vi "gentec-SOLO_PE.Read.vi"(8 "error in (no error)":errorcluster, 11 "VISA Refnum in":refnum<visa-resource-name>) -> (0 "error out":errorcluster, 1 "Return Parameters":u32[](array[numeric]), 2 "Error":string, 3 "VISA Refnum out":refnum<visa-resource-name>, 4 "Timeout":bool)   [LabVIEW 2014, in "gentec-SOLO-PE - Driver.lvlib"]
doc: "This VI tries to read out everything."
uses:
  gentec-SOLO-PE - Driver.lvlib
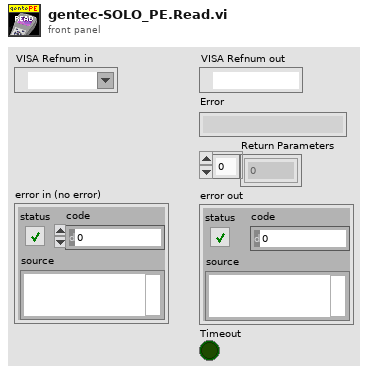
[diagram p1: front panel]
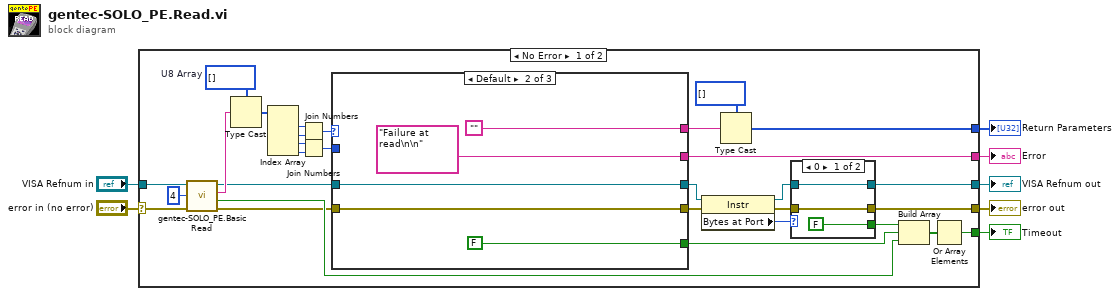
[diagram p0: block diagram]
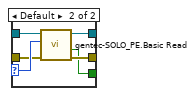
[diagram p2: hidden frame]
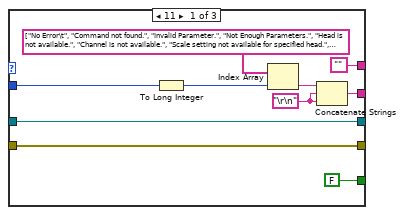
[diagram p3: hidden frame]
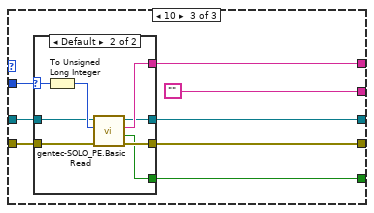
[diagram p4: hidden frame]
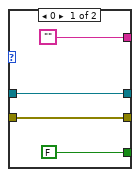
[diagram p5: hidden frame]
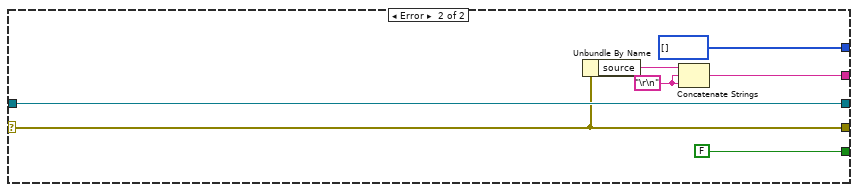
[diagram p6: hidden frame]
diagram:
  n1 = case shown="No Error" "error in (no error)" {
    selector: "error in (no error)" -> [w26 w85]
    tunnel: "VISA Refnum in" -> [w37 w86]
    tunnel: [w35 u32[] []] -> w6
    tunnel: [w19 w86] -> w5
    tunnel: [w12 w85] -> w4
    tunnel: [w16 FALSE] -> w3
    tunnel: [w23 w83] -> w2
    frame No Error {
      w36 = u8[] []  # U8 Array
      n2 = call "gentec-SOLO_PE.Basic Read.vi"("error in (no error)"=w26, "byte count"=u32 4, "VISA Refnum in"=w37) -> ("error out"=w8:errorcluster, "Timeout?"=w15:bool, "read buffer"=w33:string, "VISA Refnum out"=w9:refnum<visa-resource-name>)  [unwired: 5 in]
      n3 = Type Cast(type=w36, x=w33) -> (*(type *) &x=w28:u8[])
      n4 = Index Array(array=w28) -> (element #1=w30:u8, element #2=w29:u8, element #3=w31:u8, element #4=w32:u8)  [unwired: 4 in]
      n5 = Join Numbers(hi=w30, lo=w29) -> ((hi.lo)=w25:u16)
      n6 = Join Numbers(hi=w31, lo=w32) -> ((hi.lo)=w24:u16)
      n7 = case shown="Default" w25 {
        tunnel: [w52 "Failure at read\n\n" ("source") ""] -> w23
        tunnel: w24 -> [w53 _ w68]
        tunnel: w9 -> [w50 w60 w67]
        tunnel: [w50 w60 w66] -> w21
        tunnel: w8 -> [w49 w58 w62]
        tunnel: ["" "" w65] -> w22
        tunnel: [w49 w58 w64] -> w11
        tunnel: [FALSE ("Timeout?") FALSE ("Timeout?") w63] -> w14
        frame 11 {
          w51 = "\r\n"
          n8 = To Long Integer(number=w53) -> (32bit integer=w54:i32)
          n9 = Index Array(array=string[] ["No Error\t", "Command not found.", "Invalid Parameter.", "Not Enough Parameters.", "Head is not available.", "Channel is not available.", "Scale setting not available for specified head.", "Specified channel cannot be offset.", "No Data available.", "External trigger is not available.", "Analog output is not available.", "Anticipation is not available.", "Statistics are not available.", "Wavelength Correction is not available.", "Invalid Command: Too long.", "Too many Parameters.", "Invalid Baud Rate.", "Internal trigger is not available.", "Calorimeter mode is not available with current head."] ("Error Array"), index=w54) -> (element=w56:string)
          n10 = Concatenate Strings(w56, w51, w51) -> (w52:string)
        }
        frame Default {
        }
        frame 10 {
          n11 = case shown="Default" w68 {
            selector: w68 -> [_ w80]
            tunnel: [w72 w75] -> w64
            tunnel: ["" w81] -> w65
            tunnel: w62 -> [w72 w77]
            tunnel: w67 -> [w73 w78]
            tunnel: [w73 w76] -> w66
            tunnel: [FALSE ("Timeout?") w74] -> w63
            frame 0 {
            }
            frame Default {
              n12 = To Unsigned Long Integer(number=w80) -> (unsigned 32bit integer=w79:u32)
              n13 = call "gentec-SOLO_PE.Basic Read.vi"("error in (no error)"=w77, "byte count"=w79, "VISA Refnum in"=w78) -> ("error out"=w75:errorcluster, "Timeout?"=w74:bool, "read buffer"=w81:string, "VISA Refnum out"=w76:refnum<visa-resource-name>)  [unwired: 5 in]
            }
          }
        }
      }
      n14 = property class="Instr"(reference=w21, error in=w11) -> (reference out=w20:refnum<visa-resource-name>, error out=w13:errorcluster, "Bytes at Port"=w18:u32)
      n15 = Type Cast(type=u32[] [], x=w22) -> (*(type *) &x=w35:u32[])
      n16 = case shown="0" w18 {
        selector: w18 -> [_ w44]
        tunnel: w20 -> [w40 w46]
        tunnel: [w40 w45] -> w19
        tunnel: w13 -> [w39 w43]
        tunnel: [w39 w42] -> w12
        tunnel: [FALSE ("Timeout?") w41] -> w10
        frame 0 {
        }
        frame Default {
          n17 = call "gentec-SOLO_PE.Basic Read.vi"("error in (no error)"=w43, "byte count"=w44, "VISA Refnum in"=w46) -> ("error out"=w42:errorcluster, "Timeout?"=w41:bool, "VISA Refnum out"=w45:refnum<visa-resource-name>)  [unwired: 5 in, 1 out]
        }
      }
      n18 = Build Array(w10, w14, w15) -> (w17:bool[])
      n19 = Or Array Elements(Boolean array=w17) -> (logical OR=w16:bool)
    }
    frame Error {
      w82 = "\r\n"
      n20 = Unbundle By Name(w85) -> ("source"=w84:string)
      n21 = Concatenate Strings(w84, w82, w82) -> (w83:string)
    }
  }
  "Return Parameters" <- w6
  "error out" <- w4
  "VISA Refnum out" <- w5
  "Error" <- w2
  "Timeout" <- w3
